vi "ShowFrontPanel.vi"(8 "error in (no error)":errorcluster, 11 "Gui in":refnum<class "Gui.lvclass">) -> (0 "error out":errorcluster, 3 "Gui out":refnum<class "Gui.lvclass">)   [LabVIEW 2022 SP3, in "Gui.lvlib" / "Gui.lvclass"]
uses:
  Gui.lvclass
  Gui.lvclass/Gui.ctl
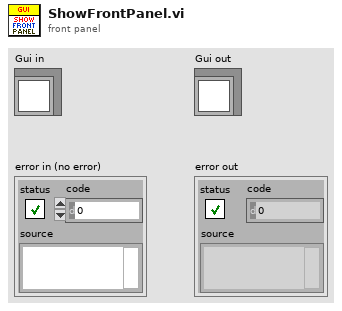
[diagram p1: front panel]
types:
  T1 = enum32{"Invalid", "Standard", "Closed", "Hidden", "Minimized", "Maximized"}
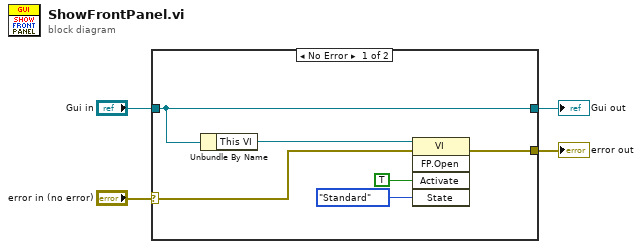
[diagram p0: block diagram]
diagram:
  n1 = case shown="No Error" "error in (no error)" {
    selector: "error in (no error)" -> [w8 w12]
    tunnel: [w7 w12] -> w3
    tunnel: [w10 w11] -> w1
    tunnel: "Gui in" -> [w10 w11]
    frame No Error {
      n2 = Unbundle By Name(w10) -> ("This VI"=w9:refnum<vi>)
      n3 = invoke class="VI" method="FP.Open"(reference=w9, error in=w8, "Activate"=TRUE ("Activate?"), "State"=T1."Standard") -> (error out=w7:errorcluster)  [unwired: 1 in, 4 out]
    }
    frame Error {
    }
  }
  "error out" <- w3
  "Gui out" <- w1
